vi "test Timeout Is Total - Not Per Item.vi"(8 "error in (no error)":errorcluster, 11 "TestCase in":refnum<class "Wait On All Future Tests.lvclass">) -> (0 "error out":errorcluster, 3 "TestCase out":refnum<class "Wait On All Future Tests.lvclass">)   [LabVIEW 2017, in "Wait On All Future Tests.lvclass"]
uses:
  Wait On All Future Tests.lvclass
  <vilib>/addons/_JKI Toolkits/VI Tester/TestCase.llb/TestCase.lvclass
  Futures/Futures.lvlib
  Futures/Future/Future.lvclass
  Futures/Promise/Promise.lvclass
  C:/Program Files (x86)/National Instruments/LabVIEW 2017/vi.lib/addons/_JKI Toolkits/VI Tester/TestCase.llb/TestCase.lvclass
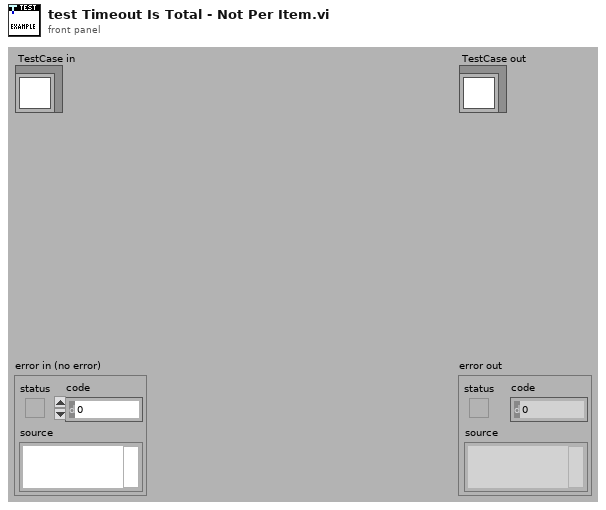
[diagram p1: front panel]
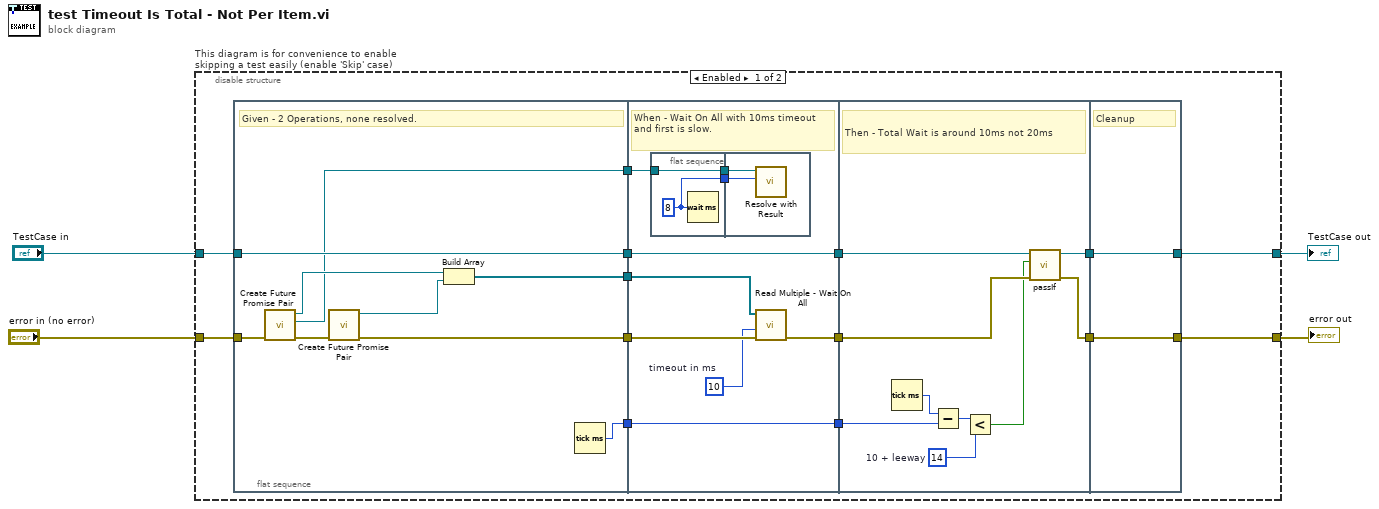
[diagram p0: block diagram]
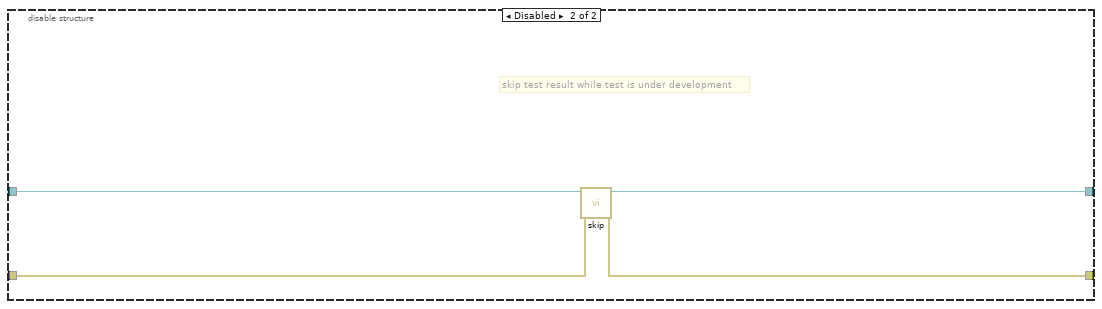
[diagram p2: hidden frame]
diagram:
  n1 = disable-structure "This diagram is for convenience to enable skipping a test easily (enable 'Skip' case)" shown="Enabled" {
    disable-tunnel: "TestCase in" -> [w14 w55]
    disable-tunnel: [w12 w53] -> w1
    disable-tunnel: [w11 w54] -> w3
    disable-tunnel: "error in (no error)" -> [w13 w52]
    frame Enabled {
      n2 = flat-sequence {
        tunnel: w13 -> [w26]
        tunnel: w14 -> [w27]
        tunnel: [w27] -> w18
        tunnel: [w21] -> w9
        tunnel: [w22] -> w8
        tunnel: [w20] -> w7
        tunnel: [w19] -> w5
        tunnel: [w36] -> w17
        tunnel: w18 -> [w36]
        tunnel: [w35] -> w10
        tunnel: w9 -> [w34]
        tunnel: w8 -> [w33]
        tunnel: w7 -> [w31]
        tunnel: [w31] -> w6
        tunnel: w5 -> [w29]
        tunnel: [w46] -> w16
        tunnel: [w44] -> w15
        tunnel: w17 -> [w47]
        tunnel: w10 -> [w45]
        tunnel: w6 -> [w48]
        tunnel: [w50] -> w11
        tunnel: [w51] -> w12
        tunnel: w16 -> [w51]
        tunnel: w15 -> [w50]
        frame #0 {
          # "Given - 2 Operations, none resolved."
          n3 = call "Create Future Promise Pair.vi"("error in (no error)"=w26) -> ("error out"=w25:errorcluster, "Promise out"=w19:refnum<class "Promise.lvclass">, "Future out"=w23:refnum<class "Future.lvclass">)  [unwired: 8 in]
          n4 = call "Create Future Promise Pair.vi"("error in (no error)"=w25) -> ("error out"=w22:errorcluster, "Future out"=w24:refnum<class "Future.lvclass">)  [unwired: 8 in, 1 out]
          n5 = Build Array(w23, w24) -> (w21:refnum<class "Future.lvclass">[])
          n6 = Tick Count (ms)() -> (millisecond timer value=w20:u32)
        }
        frame #1 {
          w32 = 10  # timeout in ms
          # "When - Wait On All with 10ms timeout and first is slow."
          n7 = flat-sequence {
            tunnel: [w38] -> w30
            tunnel: w29 -> [w37]
            tunnel: [w37] -> w28
            tunnel: w30 -> [w40]
            tunnel: w28 -> [w39]
            frame #0 {
              w38 = u32 8 ("milliseconds to wait")
              n8 = Wait (ms)(milliseconds to wait=w38) -> ()  [unwired: 1 out]
            }
            frame #1 {
              n9 = call "Resolve with Result.vi"("Result"=w40, "Promise in"=w39) -> ()  [unwired: 9 in, 1 out]
            }
          }
          n10 = call "Read Multiple - Wait On All.vi"("error in (no error)"=w33, "timeout in ms (60 sec)"=w32, "Futures in"=w34) -> ("error out"=w35:errorcluster)  [unwired: 4 in, 4 out]
        }
        frame #2 {
          w42 = u32 14  # 10 + leeway
          # "Then - Total Wait is around 10ms not 20ms"
          n11 = Tick Count (ms)() -> (millisecond timer value=w49:u32)
          n12 = Subtract(x=w49, y=w48) -> (x-y=w43:u32)
          n13 = Less?(x=w43, y=w42) -> (x < y?=w41:bool)
          n14 = call-dynamic "passIf.vi"("error in (no error)"=w45, "pass"=w41, "TestCase in"=w47) -> ("error out"=w44:errorcluster, "TestCase out"=w46:refnum<class "Wait On All Future Tests.lvclass">)  [unwired: 7 in]
        }
        frame #3 {
          # "Cleanup"
        }
      }
    }
    frame Disabled {
      # "skip test result while test is under development"
      n15 = call <vilib>:"skip.vi"("error in (no error)"=w52, "TestCase in"=w55) -> ("error out"=w54:errorcluster, "TestCase out"=w53:refnum<class "Wait On All Future Tests.lvclass">)  [unwired: 8 in]
    }
  }
  "error out" <- w3
  "TestCase out" <- w1
